vi "USB.vi"() -> ()   [LabVIEW 2014]
panel:
  in  "pH":dbl=2.0
  in  "Temp":dbl=0.037
  in  "Stop":bool
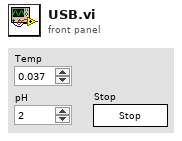
[diagram p1: front panel]
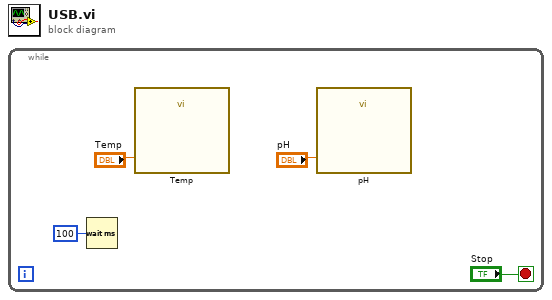
[diagram p0: block diagram]
diagram:
  n1 = while {
    stop <- "Stop" stop-if-true
    n2 = Wait (ms)(milliseconds to wait=u32 100) -> ()  [unwired: 1 out]
    n3 = call "Temp"("data"="Temp") -> ()  [unwired: 17 in, 2 out]
    n4 = call "pH"("data"="pH") -> ()  [unwired: 17 in, 2 out]
  }
